vi "TangoGroupWriteSameAttributeValueOnAllDevicesTest.vi"() -> ()   [LabVIEW 2014, in "examples.lvlib"]
uses:
  vis/tango_vi.llb/fromDoubleScalar.vi
  examples.lvlib
  vis/tango_vi.llb/tango.lvlib
panel:
  out "error out":errorcluster caption="T.Grp.W Error"
  out "attribute to write on the group":string="double_scalar"
  in  "value to write on all devices in the group":dbl=1.1
  in  "ignored devices":string[](array[string])
  in  "managed devices":string[](array[string])=["tango/tangotest/1", "tango/tangotest/2", "tango/tangotest/3"]
  in  "group name":string="w_test_group"
  out "group id":i32
  # "In this example we write the same value on all devices in the group"
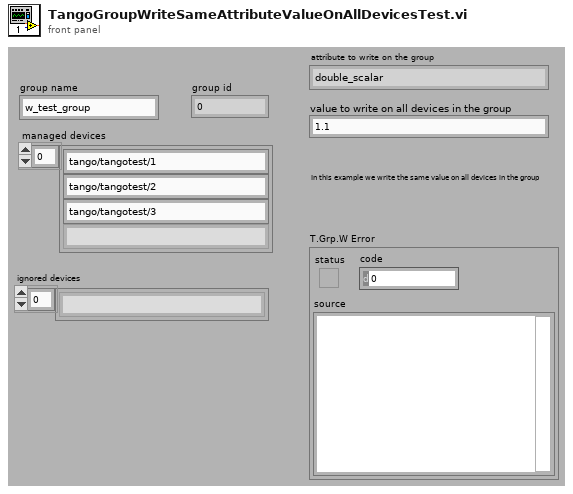
[diagram p1: front panel]
types:
  T1 = typedef "tango.lvlib/_AttributeValue_t.ctl" = cluster{"device name":string, "attribute name":string, "quality value":T2, "quality string":string, "timestamp":dbl, "dim. x":i32, "dim. y":i32, "value":u8[], "error code":i32, "error stack":string[], "data type":T3}
  T2 = typedef "tango.lvlib/_AttributeQuality_t.ctl" = enum16{"VALID", "INVALID", "ALARM", "CHANGING", "UNKNOWN_QUALITY"}
  T3 = typedef "tango.lvlib/_AttributeDataType_t.ctl" = enum16{"STATE_SCA", "STATE_SPE", "STATE_IMG", "STRING_SCA", "STRING_SPE", "STRING_IMG", "BOOL_SCA", "BOOL_SPE", "BOOL_IMG", "UCHAR_SCA", "UCHAR_SPE", "UCHAR_IMG", "SHORT_SCA", "SHORT_SPE", "SHORT_IMG", "USHORT_SCA", "USHORT_SPE", "USHORT_IMG", "LONG_SCA", "LONG_SPE", "LONG_IMG", "ULONG_SCA", "ULONG_SPE", "ULONG_IMG", "LONG64_SCA", "LONG64_SPE", "LONG64_IMG", "ULONG64_SCA", "ULONG64_SPE", "ULONG64_IMG", "FLOAT_SCA", "FLOAT_SPE", "FLOAT_IMG", "DOUBLE_SCA", "DOUBLE_SPE", "DOUBLE_IMG", "ENUM_SCA", "UNKNOWN_DATA_TYPE"}
  T4 = cluster{"device name":string, "attribute name":string, "quality value":i16, "quality string":string, "timestamp":dbl, "dim. x":i32, "dim. y":i32, "value":u8[], "error code":i32, "error stack":string[], "data type":u16}[]
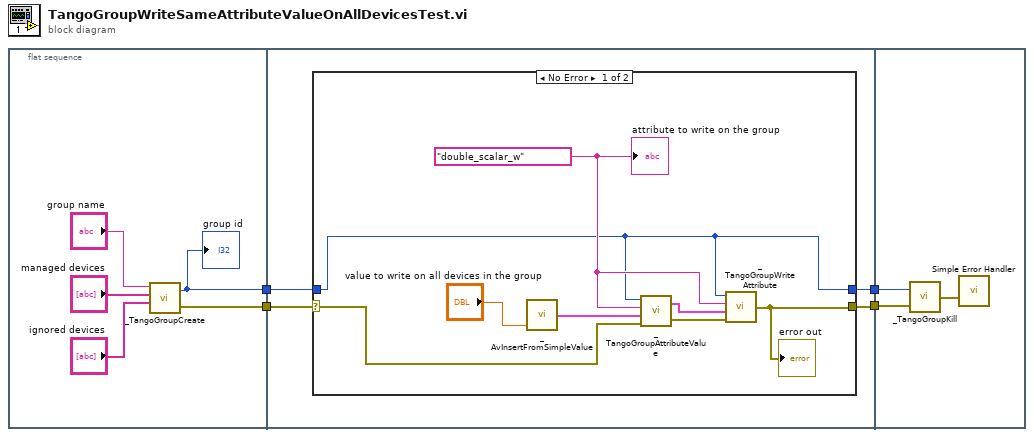
[diagram p0: block diagram]
diagram:
  n1 = flat-sequence {
    tunnel: [w8] -> w4
    tunnel: [w7] -> w3
    tunnel: w4 -> [w11]
    tunnel: [w10] -> w2
    tunnel: w3 -> [w13]
    tunnel: [w12] -> w1
    tunnel: w2 -> [w26]
    tunnel: w1 -> [w25]
    frame #0 {
      n2 = call "_TangoGroupCreate.vi"("ignored devices"="ignored devices", "managed devices"="managed devices", "group name"="group name") -> ("error out"=w7:errorcluster, "group id"=w8:i32)  [unwired: 1 in]
      "group id" <- w8
    }
    frame #1 {
      n3 = case shown="No Error" w13 {
        selector: w13 -> [w19 w23]
        tunnel: w11 -> [w17 w22]
        tunnel: [w21 w23] -> w12
        tunnel: [w17 w22] -> w10
        frame No Error {
          w18 = "double_scalar_w" ("attribute name")
          n4 = call-poly "_AvInsertFromSimpleValue.vi"("value"="value to write on all devices in the group") -> ("attribute value"=w15:T1)  [unwired: 2 in]
          n5 = call "_TangoGroupAttributeValue.vi"("error in"=w19, "attribute value"=w15, "attribute name"=w18, "group id"=w17) -> ("error out"=w20:errorcluster, "attributes_values"=w14:T4)
          n6 = call "_TangoGroupWriteAttribute.vi"("error in"=w20, "values"=w14, "attribute name"=w18, "group id"=w17) -> ("error out"=w21:errorcluster)
          "error out" <- w21
          "attribute to write on the group" <- w18
        }
        frame Error {
        }
      }
    }
    frame #2 {
      n7 = call "_TangoGroupKill.vi"("error in"=w25, "group id"=w26) -> ("error out"=w24:errorcluster)
      n8 = call <vilib>:"Simple Error Handler.vi"("error in (no error)"=w24) -> ()  [unwired: 4 in, 5 out]
    }
  }
